vi "Read Step Data (DC Parallel Manual Mode).vi"   [LabVIEW 2016, in "APT 300XAC Series.lvlib"]
doc: "Read the step data being displayed on the LCD display while the test is in process. Parallel Manual Mode only."
uses:
  APT 300XAC Series.lvlib
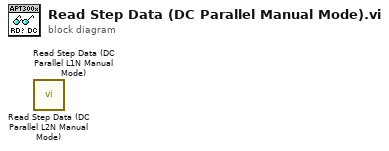
[diagram p0: block diagram]
diagram:
  n1 = call "Read Step Data (DC Parallel L2N Manual Mode).vi"() -> ()  [unwired: 13 in, 3 out]
  n2 = call "Read Step Data (DC Parallel L1N Manual Mode).vi"() -> ()  [unwired: 13 in, 3 out]
